vi "getEnd.vi"(0 "reference":refnum<class "AbstractEdge.lvclass">, 5 "error in (no error)":errorcluster) -> (14 "reference out":refnum<class "AbstractEdge.lvclass">, 15 "endNode":refnum<class "AbstractNode.lvclass">, 16 "validNode":bool, 19 "error out":errorcluster)   [LabVIEW 2016, in "AbstractEdge.lvclass"]
doc: "public Node getEnd()"
uses:
  <resource>/Framework/Providers/Open_GDS/UML/AbstractEdge_class/AbstractEdge.lvclass
  <resource>/Framework/Providers/Open_GDS/UML/AbstractNode_class/AbstractNode.lvclass
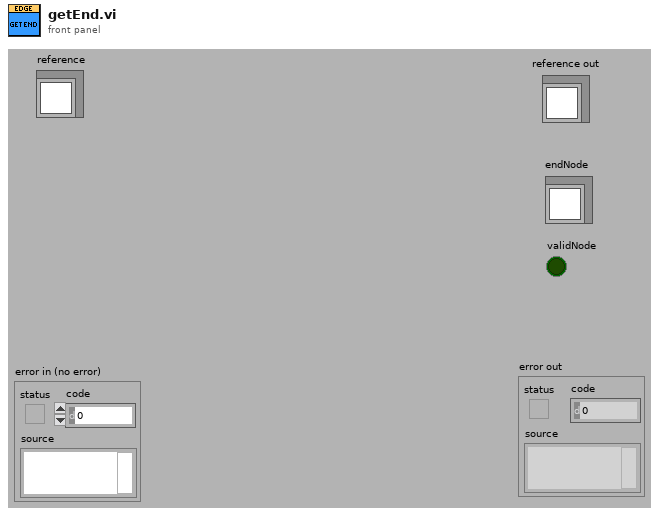
[diagram p1: front panel]
types:
  T1 = typedef "AbstractEdge.lvclass/ObjectAttributes.ctl" = cluster{"start":refnum<class "AbstractNode.lvclass">, "end":refnum<class "AbstractNode.lvclass">}
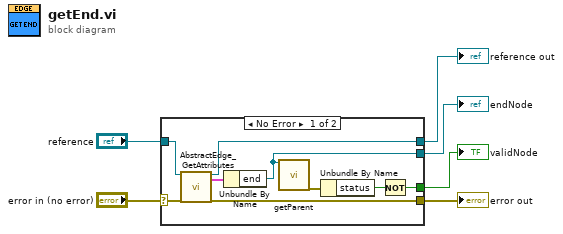
[diagram p0: block diagram]
diagram:
  n1 = case shown="No Error" "error in (no error)" {
    selector: "error in (no error)" -> [w12 w16]
    tunnel: "reference" -> [w15 w17]
    tunnel: [w14 w16] -> w5
    tunnel: [w13 w17] -> w4
    tunnel: [w8 _] -> w2
    tunnel: [w11 _] -> w1
    frame No Error {
      n2 = call <resource>:"AbstractEdge_GetAttributes.vi"("reference in"=w15, "error in (no error)"=w12) -> ("reference out"=w13:refnum<class "AbstractEdge.lvclass">, "Data"=w7:T1, "error out"=w14:errorcluster)  [unwired: 1 in, 14 out]
      n3 = Unbundle By Name(w7) -> ("end"=w11:refnum<class "AbstractNode.lvclass">)
      n4 = call-dynamic "getParent.vi"("reference"=w11) -> ("error out"=w10:errorcluster)  [unwired: 14 in, 4 out]
      n5 = Unbundle By Name(w10) -> ("status"=w9:bool)
      n6 = Not(x=w9) -> (.not. x?=w8:bool)
    }
    frame Error {
    }
  }
  "reference out" <- w4
  "error out" <- w5
  "endNode" <- w1
  "validNode" <- w2
